vi "Wav_Analyzer.vi"(8 "error in (no error)":errorcluster, 9 "Wavelet":u16(ring) items=["db02"=0, "db03"=1, "db04"=2, "db05"=3, "db06"=4, "db07"=5, "db08"=6, "db09"=7, "db10"=8, "db11"=9, "db12"=10, "db13"=11, "db14"=12, "Haar"=13, "bior1_3"=14, "bior1_5"=15, "bior2_2"=16, "bior2_4"=17, "bior2_6"=18, "bior2_8"=19, "bior3_1"=20, "bior3_3"=21, "bior3_5"=22, "bior3_7"=23, "bior3_9"=24, "bior4_4 (FBI)"=25, "bior5_5"=38, "bior6_8"=39, "coif1"=26, "coif2"=27, "coif3"=28, "coif4"=29, "coif5"=30, "sym2"=31, "sym3"=32, "sym4"=33, "sym5"=34, "sym6"=35, "sym7"=36, "sym8"=37], 10 "Decomposition Level":i32=1 min=1 step=1, 11 "DataIn":T1) -> (0 "error out":errorcluster)   [LabVIEW 2012]
doc: "VI decomposes given signal with selected wavelet and to specified level."
uses:
  Signal/#TD_SignalStorageData.ctl
  Signal/#TD_SignalStorageCommand.ctl
  <vilib>/addons/Wavelet Analysis/filter banks.llb/WA 1D Analysis Filter Bank (Waveform).vi
  <vilib>/addons/_Advanced Signal Processing/NI_AdvSigProcWA.lvlib
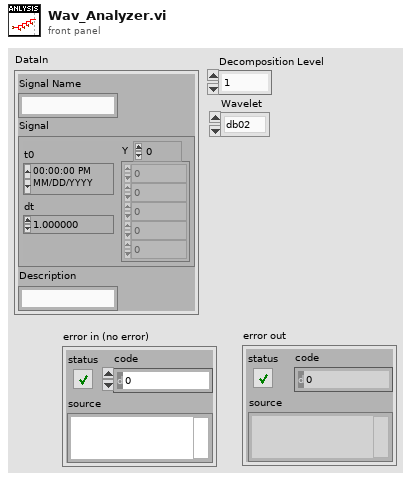
[diagram p1: front panel]
types:
  T1 = typedef "#TD_SignalStorageData.ctl" = cluster{"Signal Name":string, "Signal":waveform(dbl), "Description":string}
  T2 = typedef "#TD_SignalStorageCommand.ctl" = enum16{"Reset_Storage", "Add_Signal", "Insert_Signal", "Del_Signal", "Replace_Signal", "Get_Signal", "Get_Signal_List", "Change_Signal_Name", "Change_Signal_Descr"}
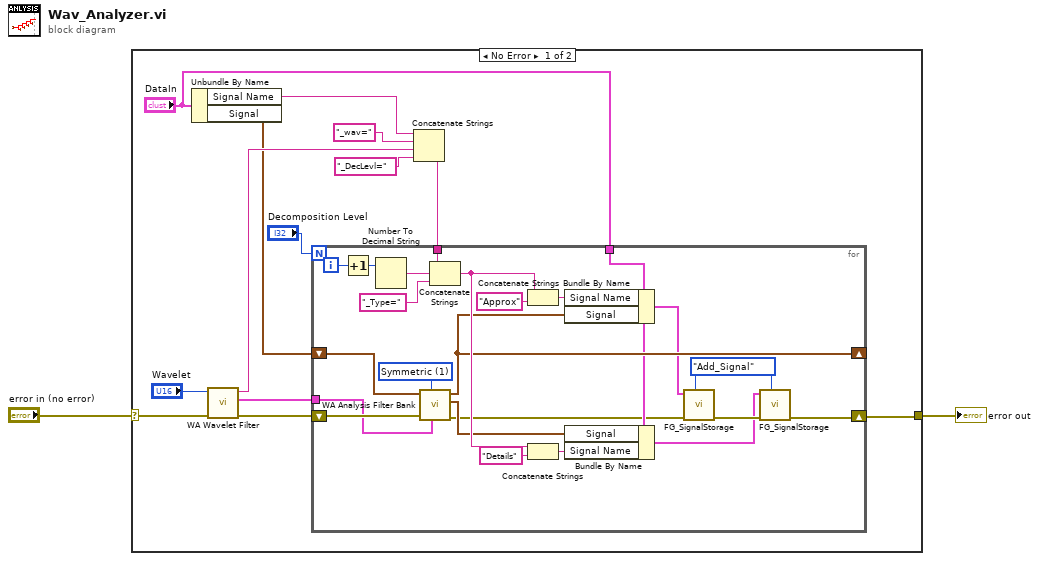
[diagram p0: block diagram]
diagram:
  n1 = case shown="No Error" "error in (no error)" {
    selector: "error in (no error)" -> [w14 w39]
    tunnel: [w3 w39] -> w1
    frame No Error {
      n2 = Unbundle By Name("DataIn") -> ("Signal Name"=w6:string, "Signal"=w5:waveform(dbl))
      n3 = call <vilib>:"WA Wavelet Filter.vi"("error in (no error)"=w14, "wavelet"="Wavelet") -> ("error out"=w13:errorcluster, "analysis filters"=w12:cluster{"lowpass":dbl[], "highpass":dbl[]}, "wavelet name"=w8:string)  [unwired: 6 in, 1 out]
      n4 = Concatenate Strings(w6, "_wav=" ("string"), w8, "_DecLevl=" ("string")) -> (w7:string)
      n5 = for {
        N: "Decomposition Level" -> [_]
        tunnel: w12 -> [w34]
        shift-right: [w26] -> _
        shift-left: w5 -> [w36]
        tunnel: w7 -> [w32]
        tunnel: "DataIn" -> [w25]
        shift-right: [w20] -> w3
        shift-left: w13 -> [w37]
        i -> [w33]
        w17 = #TD_SignalStorageCommand."Add_Signal" ("Command")
        w35 = u16 1 items=["Zero padding", "Symmetric", "Periodic"] ("extension")
        n6 = Increment(x=w33) -> (x+1=w16:i32)
        n7 = Number To Decimal String(number=w16) -> (decimal integer string=w31:string)  [unwired: 1 in]
        n8 = call-poly <vilib>:"WA Analysis Filter Bank.vi"("analysis filters"=w34, "extension"=w35, "error in (no error)"=w37, "signal"=w36) -> ("error out"=w22:errorcluster, "detail coef"=w24:waveform(dbl), "approx coef"=w26:waveform(dbl))  [unwired: 5 in]
        n9 = Concatenate Strings(w32, w31, "_Type=" ("string")) -> (w38:string)
        n10 = Concatenate Strings(w38, "Approx" ("string")) -> (w27:string)
        n11 = Concatenate Strings(w38, "Details" ("string")) -> (w23:string)
        n12 = Bundle By Name(cluster=w25, "Signal Name"=w27, "Signal"=w26) -> (w19:T1)
        n13 = Bundle By Name(cluster=w25, "Signal"=w24, "Signal Name"=w23) -> (w18:T1)
        n14 = call "FG_SignalStorage.vi"("Command"=w17, "error in (no error)"=w22, "DataIn"=w19) -> ("error out"=w21:errorcluster)  [unwired: 6 in, 2 out]
        n15 = call "FG_SignalStorage.vi"("Command"=w17, "error in (no error)"=w21, "DataIn"=w18) -> ("error out"=w20:errorcluster)  [unwired: 6 in, 2 out]
      }
    }
    frame Error {
    }
  }
  "error out" <- w1
